vi "Create Timing.vi"(6 "priority":u64, 7 "id (0)":i32, 8 "error in (no error)":errorcluster, 9 "offset":u64, 10 "decimation":u64=1, 11 "Timing in":refnum<class "Timing.lvclass">) -> (0 "error out":errorcluster, 3 "Timing out":refnum<class "Timing.lvclass">)   [LabVIEW 2021, in "DSF Core.lvlib" / "Timing.lvclass"]
uses:
  Timing.lvclass
  Timing.lvclass/Timing.ctl
  Invalid Priority.vi
  Invalid Offset.vi
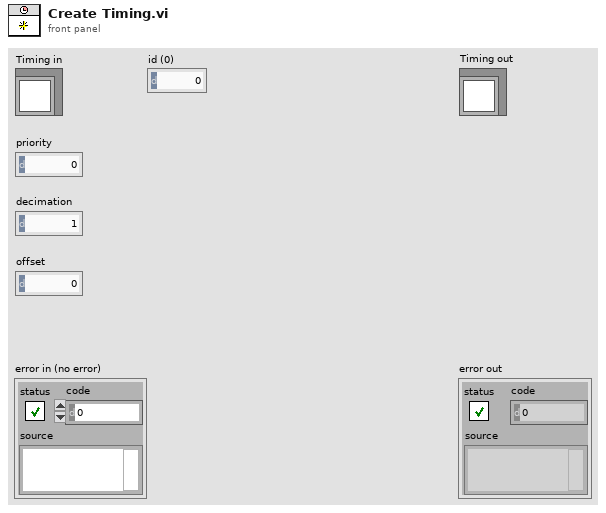
[diagram p1: front panel]
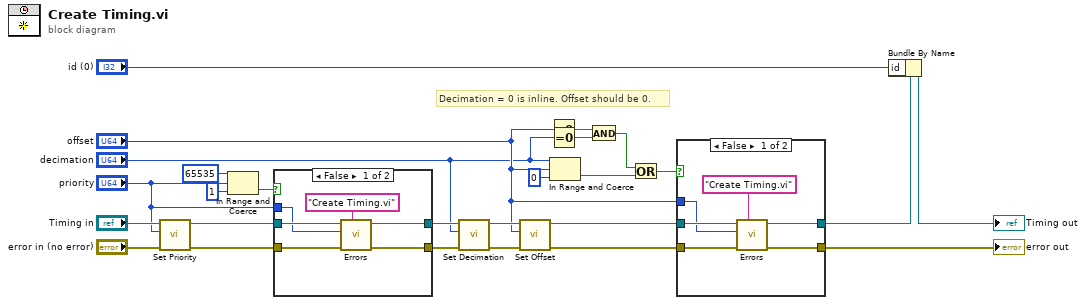
[diagram p0: block diagram]
diagram:
  # "Decimation = 0 is inline. Offset should be 0."
  n1 = call "Set Priority.vi"("Priority"="priority", "Timing in"="Timing in") -> ("Timing out"=w12:refnum<class "Timing.lvclass">)  [unwired: 9 in]
  n2 = In Range and Coerce(upper limit=u64 65535, x="priority", lower limit=u64 1) -> (In Range?=w5:bool)  [unwired: 1 out]
  n3 = case shown="False" w5 {
    tunnel: w12 -> [w29 w31]
    tunnel: [w28 w31] -> w11
    tunnel: "error in (no error)" -> [w27 w30]
    tunnel: [w26 w30] -> w9
    tunnel: "priority" -> [w24 _]
    frame False {
      n4 = call-poly "Errors.vi"("error source vi name"="Create Timing.vi", "error in (no error)"=w27, "priority"=w24, "Timing in"=w29) -> ("error out"=w26:errorcluster, "Timing out"=w28:refnum<class "Timing.lvclass">)  [unwired: 6 in]
    }
    frame True {
    }
  }
  n5 = call "Set Decimation.vi"("Decimation"="decimation", "Timing in"=w11) -> ("Timing out"=w22:refnum<class "Timing.lvclass">)  [unwired: 9 in]
  n6 = call "Set Offset.vi"("Offset"="offset", "Timing in"=w22) -> ("Timing out"=w20:refnum<class "Timing.lvclass">)  [unwired: 9 in]
  n7 = Equal To 0?(x="offset") -> (x = 0?=w16:bool)
  n8 = Equal To 0?(x="decimation") -> (x = 0?=w17:bool)
  n9 = In Range and Coerce(upper limit="decimation", x="offset", lower limit=u64 0) -> (In Range?=w15:bool)  [unwired: 1 out]
  n10 = And(x=w16, y=w17) -> (x .and. y?=w13:bool)
  n11 = Or(x=w13, y=w15) -> (x .or. y?=w14:bool)
  n12 = case shown="False" w14 {
    tunnel: w20 -> [w37 w39]
    tunnel: [w36 w39] -> w2
    tunnel: [w35 w38] -> w19
    tunnel: w9 -> [w34 w38]
    tunnel: "offset" -> [w33 _]
    frame False {
      n13 = call-poly "Errors.vi"("error source vi name"="Create Timing.vi", "error in (no error)"=w34, "offset"=w33, "Timing in"=w37) -> ("error out"=w35:errorcluster, "Timing out"=w36:refnum<class "Timing.lvclass">)  [unwired: 6 in]
    }
    frame True {
    }
  }
  "error out" <- w19
  n14 = Bundle By Name(cluster=w2, "id"="id (0)") -> (→"Timing out":refnum<class "Timing.lvclass">)
